vi "Render.vi"(7 "Renderer":refnum<class "Renderer.lvclass">, 8 "error in (no error)":errorcluster, 10 "Camera":refnum<class "Camera.lvclass">, 11 "Slylandro in":refnum<class "Slylandro.lvclass">) -> (0 "error out":errorcluster)   [LabVIEW 2026]
uses:
  Slylandro.lvclass
  Camera/Camera.lvclass
  Renderer/Renderer.lvclass
  Slylandro.lvclass/Slylandro.ctl
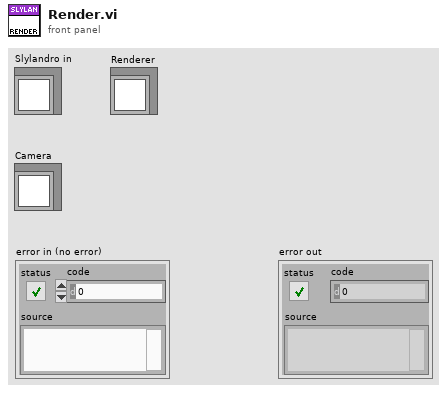
[diagram p1: front panel]
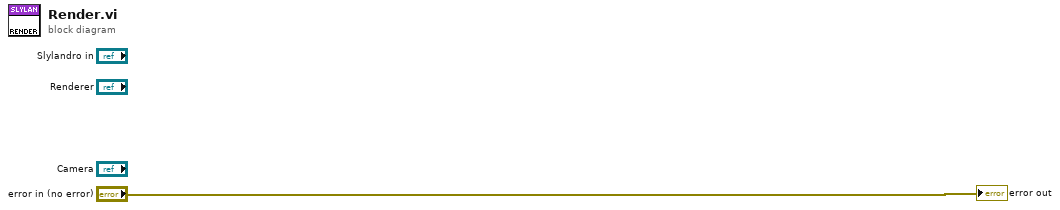
[diagram p0: block diagram]
diagram:
  "error out" <- "error in (no error)"
